vi "Get Config String.vi"(11 "Assert Add Configuration":T1) -> (3 "Case":string)   [LabVIEW 2018]
uses:
  Assert Add Configuration.ctl
  Inline or Forked.ctl
  0f10d11f-dd57-486a-8ebf-afa8c80eb204.vi
  <vilib>/JDP Science/JSONtext/Find Item.vi
  0f10d11f-dd57-486a-8ebf-afa8c80eb204.vi/80627bcc-be53-4f02-8b41-cc1d1c91fd36.vi
  <vilib>/JDP Science/JSONtext/String Subset.vi
  Wizard Config/Wizard Strings.vi
  Wizard Config/Create Default Wizard Configuration.vi
  <vilib>/JDP Science/JSONtext/Parsing/Parse Full Path or Item Name.vi
  <vilib>/JDP Science/JSONtext/Offset/Find Item Locations by Path.vi
  <vilib>/JDP Science/JSONtext/JSON text to Variant.vi
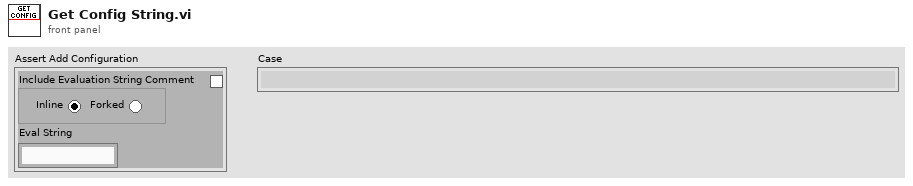
[diagram p1: front panel]
types:
  T1 = typedef "Assert Add Configuration.ctl" = cluster{"Include Evaluation String Comment":bool, "Inline or Forked":T2, "Eval String":string}
  T2 = typedef "Inline or Forked.ctl" = enum32{"Inline", "Forked"}
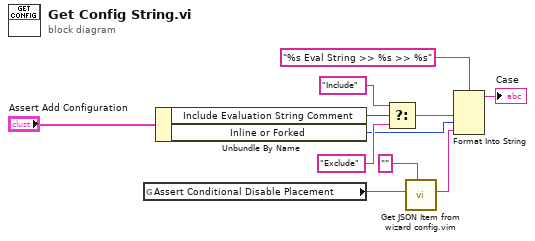
[diagram p0: block diagram]
diagram:
  n1 = global read "Wizard Strings.vi" "Assert Conditional Disable Placement"() -> (w2:string)
  n2 = Unbundle By Name("Assert Add Configuration") -> ("Include Evaluation String Comment"=w9:bool, "Inline or Forked"=w5:T2)
  n3 = Select(t="Include" ("format string"), s=w9, f="Exclude" ("format string")) -> (s? t:f=w6:string)
  n4 = call "Get JSON Item from wizard config.vim"("Data Type"="" ("$Path or Item Name"), "$Path or Item Name"=w2) -> ("<JSON>"=w1:string)  [unwired: 7 in, 2 out]
  n5 = Format Into String(format string="%s Eval String >> %s >> %s", w6, w5, w1) -> (resulting string=→"Case":string)  [unwired: 2 in, 1 out]
